vi "Drive Straight.vi"(3 "reinitialize? (F)":bool, 4 "Maneuver":T1(ring), 5 "Turn Setpoint":dbl, 6 "Drive Setpoint":dbl, 7 "Angle":dbl, 8 "Angle to Get":dbl, 9 "Enable?":bool) -> (1 "Turn Setpoint":dbl)   [LabVIEW 2018]
uses:
  <vilib>/addons/control/pid/pid.llb/PID (DBL).vi
  <vilib>/addons/control/pid/NI_PID_pid.lvlib
panel:
  out "Waveform Chart 2":cluster{"Angle to Get":dbl}(graph)
  out "Waveform Chart":cluster{dbl, dbl}(graph)
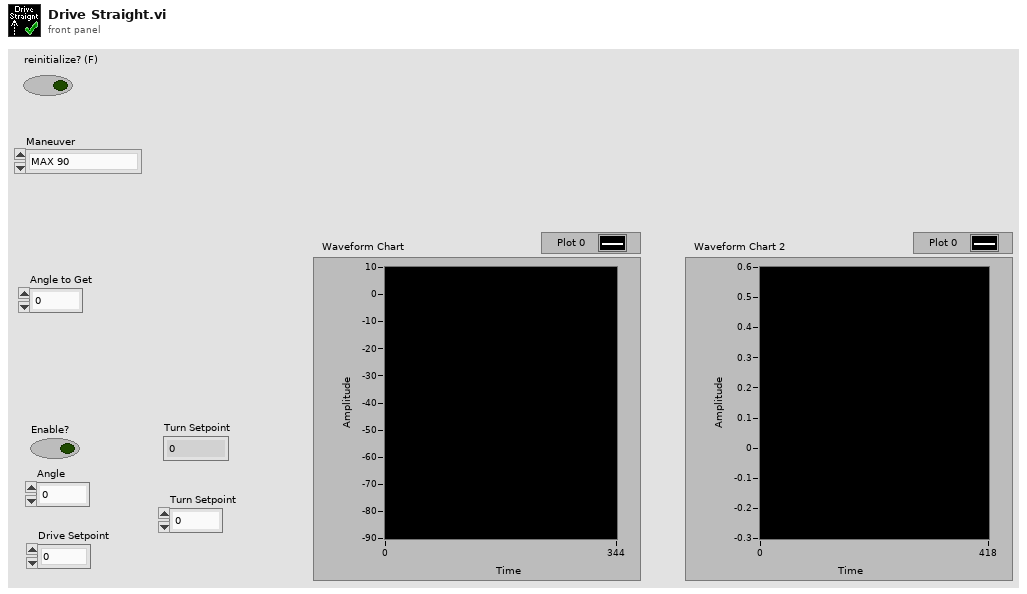
[diagram p1: front panel]
types:
  T1 = enum16{"MAX 90", "MAX 180", "Turn to Home", "Turn to Rocket", "Auto-Align", "Turn to ..."}
  T2 = cluster{"proportional gain (Kc)":dbl, "integral time (Ti, min)":dbl, "derivative time (Td, min)":dbl}
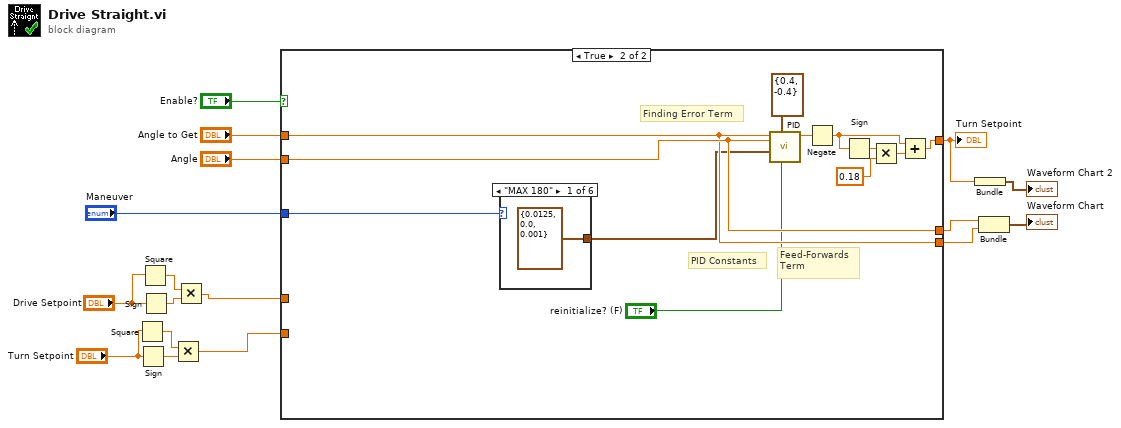
[diagram p0: block diagram]
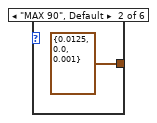
[diagram p3: hidden frame]
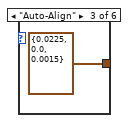
[diagram p4: hidden frame]
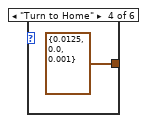
[diagram p5: hidden frame]
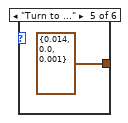
[diagram p6: hidden frame]
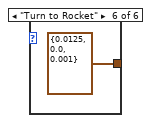
[diagram p7: hidden frame]
diagram:
  n1 = Square(x="Turn Setpoint") -> (x^2=w13:dbl)
  n2 = Sign(1:"Turn Setpoint") -> (0:w12:dbl)
  n3 = Square(x="Drive Setpoint") -> (x^2=w10:dbl)
  n4 = Sign(1:"Drive Setpoint") -> (0:w9:dbl)
  n5 = Multiply(x=w13, y=w12) -> (x*y=w11:dbl)
  n6 = Multiply(x=w10, y=w9) -> (x*y=w8:dbl)
  n7 = case shown="True" "Enable?" {
    tunnel: [w18 w20] -> w2
    tunnel: "Angle" -> [_ w29]
    tunnel: w8 -> [_ _]
    tunnel: "Angle to Get" -> [_ w28]
    tunnel: w11 -> [w18 _]
    tunnel: [_ w29] -> w4
    tunnel: [_ w28] -> w3
    tunnel: "Maneuver" -> [_ w26]
    frame False {
    }
    frame True {
      # "Feed-Forwards\nTerm"
      # "PID Constants"
      # "Finding Error Term"
      n8 = case shown="\"MAX 180\"" w26 {
        tunnel: [T2 {"proportional gain (Kc)"=0.0125, "integral time (Ti, min)"=0.0, "derivative time (Td, min)"=0.001} ("PID gains M") T2 {"proportional gain (Kc)"=0.0125, "integral time (Ti, min)"=0.0, "derivative time (Td, min)"=0.001} ("PID gains M") T2 {"proportional gain (Kc)"=0.0225, "integral time (Ti, min)"=0.0, "derivative time (Td, min)"=0.0015} ("PID gains M") T2 {"proportional gain (Kc)"=0.0125, "integral time (Ti, min)"=0.0, "derivative time (Td, min)"=0.001} ("PID gains M") T2 {"proportional gain (Kc)"=0.014, "integral time (Ti, min)"=0.0, "derivative time (Td, min)"=0.001} ("PID gains M") T2 {"proportional gain (Kc)"=0.0125, "integral time (Ti, min)"=0.0, "derivative time (Td, min)"=0.001} ("PID gains M")] -> w25
        frame "MAX 180" {
        }
        frame "MAX 90", Default {
        }
        frame "Auto-Align" {
        }
        frame "Turn to Home" {
        }
        frame "Turn to ..." {
        }
        frame "Turn to Rocket" {
        }
      }
      n9 = call-poly <vilib>:"PID.vi"("reinitialize? (F)"="reinitialize? (F)", "output range"=cluster{"output high":dbl, "output low":dbl} {"output high"=0.4, "output low"=-0.4}, "PID gains"=w25, "process variable"=w29, "setpoint"=w28) -> ("output"=w24:dbl)  [unwired: 5 in, 1 out]
      n10 = Negate(x=w24) -> (-x=w21:dbl)
      n11 = Sign(1:w21) -> (0:w23:dbl)
      n12 = Multiply(x=w23, y=0.18) -> (x*y=w22:dbl)
      n13 = Add(x=w21, y=w22) -> (x+y=w20:dbl)
    }
  }
  "Turn Setpoint" <- w2
  n14 = Bundle(w2) -> (→"Waveform Chart 2":cluster{dbl})  [unwired: 1 in]
  n15 = Bundle("Angle"=w4, "Angle to Get"=w3) -> (→"Waveform Chart":cluster{"Angle":dbl, "Angle to Get":dbl})  [unwired: 1 in]
